vi "obtain_latest_instance_from_TLC_type.vi"(8 "error in (no error)":errorcluster, 11 "top-level component type":T1) -> (0 "error out":errorcluster, 3 "GenericToplevelComponent.lvclass":refnum<class "GenericToplevelComponent.lvclass">)   [LabVIEW 2010, in "GenericToplevelComponent.lvclass"]
uses:
  GenericToplevelComponent.lvclass
  enumerations/top-level_component_type_enum.ctl
  components/ImagingMode/GenericImagingMode/GenericImagingMode/GenericImagingMode.lvclass
  components/ScanHead/GenericScanHead/GenericScanHead/GenericScanHead.lvclass
  components/DAQ/GenericDAQ/GenericDAQ/GenericDAQ.lvclass
  components/ImageAssembler/GenericImageAssembler/GenericImageAssembler/GenericImageAssembler.lvclass
  components/Display/GenericDisplay/GenericDisplay/GenericDisplay.lvclass
  components/DataCollection/GenericDataCollection/GenericDataCollection/GenericDataCollection.lvclass
  components/Analyser/GenericAnalyser/GenericAnalyser/GenericAnalyser.lvclass
  components/Stimulator/GenericStimulator/GenericStimulator/GenericStimulator.lvclass
  components/ExperimentController/GenericExperimentController/GenericExperimentController/GenericExperimentController.lvclass
  components/Instrument/GenericInstrument/GenericInstrument/GenericInstrument.lvclass
  components/Stage/GenericStage/GenericStage/GenericStage.lvclass
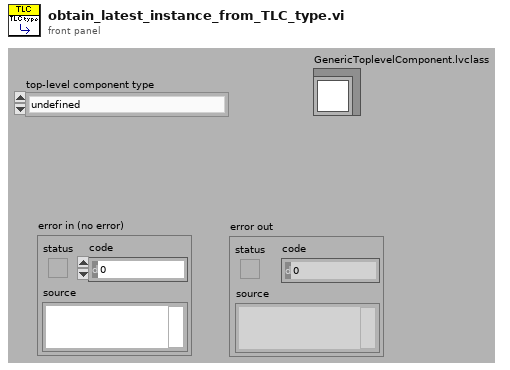
[diagram p1: front panel]
types:
  T1 = typedef "top-level_component_type_enum.ctl" = enum16{"undefined", "ImagingMode", "ScanHead", "DAQ", "ImageAssembler", "Display", "DataCollection", "Analyser", "Stimulator", "ExperimentController", "Instrument", "Stage"}
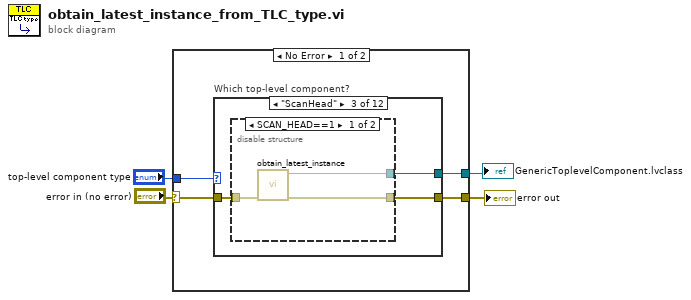
[diagram p0: block diagram]
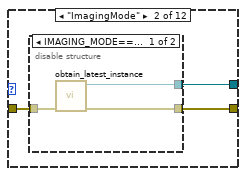
[diagram p3: hidden frame]
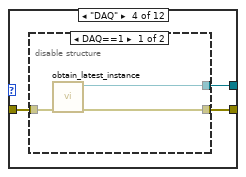
[diagram p6: hidden frame]
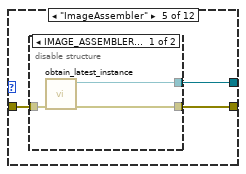
[diagram p8: hidden frame]
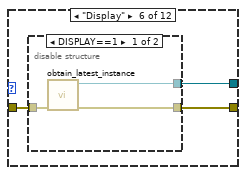
[diagram p10: hidden frame]
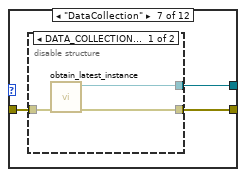
[diagram p12: hidden frame]
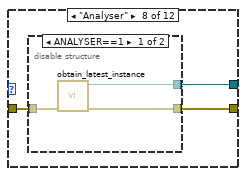
[diagram p14: hidden frame]
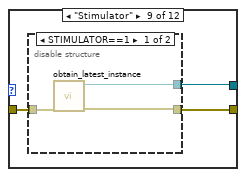
[diagram p16: hidden frame]
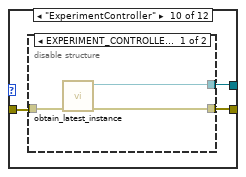
[diagram p18: hidden frame]
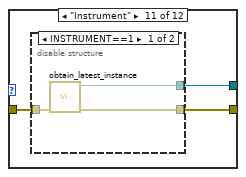
[diagram p20: hidden frame]
diagram:
  n1 = case shown="No Error" "error in (no error)" {
    selector: "error in (no error)" -> [w8 w87]
    tunnel: [w7 w87] -> w3
    tunnel: "top-level component type" -> [w6 _]
    tunnel: [w5 _] -> w1
    frame No Error {
      n2 = case "Which top-level component?" shown="\"ScanHead\"" w6 {
        tunnel: [w9 w11 w18 w25 w32 w39 w46 w53 w60 w67 w74 w81] -> w7
        tunnel: w8 -> [w9 w12 w19 w26 w33 w40 w47 w54 w61 w68 w75 w82]
        tunnel: [_ w10 w17 w24 w31 w38 w45 w52 w59 w66 w73 w80] -> w5
        frame "undefined", Default {
        }
        frame "ImagingMode" {
          n3 = disable-structure shown="IMAGING_MODE==1" {
            disable-tunnel: w12 -> [w15 w16]
            disable-tunnel: [w13 w16] -> w11
            disable-tunnel: [w14 _] -> w10
            frame condition #0 {
              n4 = call "obtain_latest_instance.vi"("error in (no error)"=w15) -> ("error out"=w13:errorcluster, "GenericScanMode out"=w14:refnum<class "GenericImagingMode.lvclass">)  [unwired: 9 in]
            }
            frame condition #1 (active) {
            }
          }
        }
        frame "ScanHead" {
          n5 = disable-structure shown="SCAN_HEAD==1" {
            disable-tunnel: w19 -> [w22 w23]
            disable-tunnel: [w21 w23] -> w18
            disable-tunnel: [w20 _] -> w17
            frame condition #0 {
              n6 = call "obtain_latest_instance.vi"("error in (no error)"=w22) -> ("error out"=w21:errorcluster, "GenericScanHead out"=w20:refnum<class "GenericScanHead.lvclass">)  [unwired: 9 in]
            }
            frame condition #1 (active) {
            }
          }
        }
        frame "DAQ" {
          n7 = disable-structure shown="DAQ==1" {
            disable-tunnel: w26 -> [w29 w30]
            disable-tunnel: [w27 w30] -> w25
            disable-tunnel: [w28 _] -> w24
            frame condition #0 {
              n8 = call "obtain_latest_instance.vi"("error in (no error)"=w29) -> ("error out"=w27:errorcluster, "GenericDAQ out"=w28:refnum<class "GenericDAQ.lvclass">)  [unwired: 9 in]
            }
            frame condition #1 (active) {
            }
          }
        }
        frame "ImageAssembler" {
          n9 = disable-structure shown="IMAGE_ASSEMBLER==1" {
            disable-tunnel: w33 -> [w36 w37]
            disable-tunnel: [w34 w37] -> w32
            disable-tunnel: [w35 _] -> w31
            frame condition #0 {
              n10 = call "obtain_latest_instance.vi"("error in (no error)"=w36) -> ("error out"=w34:errorcluster, "GenericImageAssembler out"=w35:refnum<class "GenericImageAssembler.lvclass">)  [unwired: 9 in]
            }
            frame condition #1 (active) {
            }
          }
        }
        frame "Display" {
          n11 = disable-structure shown="DISPLAY==1" {
            disable-tunnel: w40 -> [w43 w44]
            disable-tunnel: [w42 w44] -> w39
            disable-tunnel: [w41 _] -> w38
            frame condition #0 {
              n12 = call "obtain_latest_instance.vi"("error in (no error)"=w43) -> ("error out"=w42:errorcluster, "GenericDisplay out"=w41:refnum<class "GenericDisplay.lvclass">)  [unwired: 9 in]
            }
            frame condition #1 (active) {
            }
          }
        }
        frame "DataCollection" {
          n13 = disable-structure shown="DATA_COLLECTION==1" {
            disable-tunnel: w47 -> [w50 w51]
            disable-tunnel: [w48 w51] -> w46
            disable-tunnel: [w49 _] -> w45
            frame condition #0 {
              n14 = call "obtain_latest_instance.vi"("error in (no error)"=w50) -> ("error out"=w48:errorcluster, "GenericDataCollection out"=w49:refnum<class "GenericDataCollection.lvclass">)  [unwired: 9 in]
            }
            frame condition #1 (active) {
            }
          }
        }
        frame "Analyser" {
          n15 = disable-structure shown="ANALYSER==1" {
            disable-tunnel: w54 -> [w57 w58]
            disable-tunnel: [w56 w58] -> w53
            disable-tunnel: [w55 _] -> w52
            frame condition #0 {
              n16 = call "obtain_latest_instance.vi"("error in (no error)"=w57) -> ("error out"=w56:errorcluster, "GeneralAnalyser out"=w55:refnum<class "GenericAnalyser.lvclass">)  [unwired: 9 in]
            }
            frame condition #1 (active) {
            }
          }
        }
        frame "Stimulator" {
          n17 = disable-structure shown="STIMULATOR==1" {
            disable-tunnel: w61 -> [w64 w65]
            disable-tunnel: [w62 w65] -> w60
            disable-tunnel: [w63 _] -> w59
            frame condition #0 {
              n18 = call "obtain_latest_instance.vi"("error in (no error)"=w64) -> ("error out"=w62:errorcluster, "GenericStimulator out"=w63:refnum<class "GenericStimulator.lvclass">)  [unwired: 9 in]
            }
            frame condition #1 (active) {
            }
          }
        }
        frame "ExperimentController" {
          n19 = disable-structure shown="EXPERIMENT_CONTROLLER==1" {
            disable-tunnel: w68 -> [w71 w72]
            disable-tunnel: [w69 w72] -> w67
            disable-tunnel: [w70 _] -> w66
            frame condition #0 {
              n20 = call "obtain_latest_instance.vi"("error in (no error)"=w71) -> ("error out"=w69:errorcluster, "GenericExperimentController out"=w70:refnum<class "GenericExperimentController.lvclass">)  [unwired: 9 in]
            }
            frame condition #1 (active) {
            }
          }
        }
        frame "Instrument" {
          n21 = disable-structure shown="INSTRUMENT==1" {
            disable-tunnel: w75 -> [w78 w79]
            disable-tunnel: [w77 w79] -> w74
            disable-tunnel: [w76 _] -> w73
            frame condition #0 {
              n22 = call "obtain_latest_instance.vi"("error in (no error)"=w78) -> ("error out"=w77:errorcluster, "microscope"=w76:refnum<class "GenericInstrument.lvclass">)  [unwired: 9 in]
            }
            frame condition #1 (active) {
            }
          }
        }
        frame "Stage" {
          n23 = disable-structure shown="STAGE==1" {
            disable-tunnel: w82 -> [w85 w86]
            disable-tunnel: [w83 w86] -> w81
            disable-tunnel: [w84 _] -> w80
            frame condition #0 {
              n24 = call "obtain_latest_instance.vi"("error in (no error)"=w85) -> ("error out"=w83:errorcluster, "GenericStage out"=w84:refnum<class "GenericStage.lvclass">)  [unwired: 9 in]
            }
            frame condition #1 (active) {
            }
          }
        }
      }
    }
    frame Error {
    }
  }
  "GenericToplevelComponent.lvclass" <- w1
  "error out" <- w3
